vi "TImeThresholdLogic(SubVI).vi"(2 "Position":dbl[](array[numeric]), 3 "Bits":dbl[](array[numeric]), 4 "Buffer":dbl[][](array[numeric])) -> (0 "Data":dbl[][](array[numeric]))   [LabVIEW 2017]
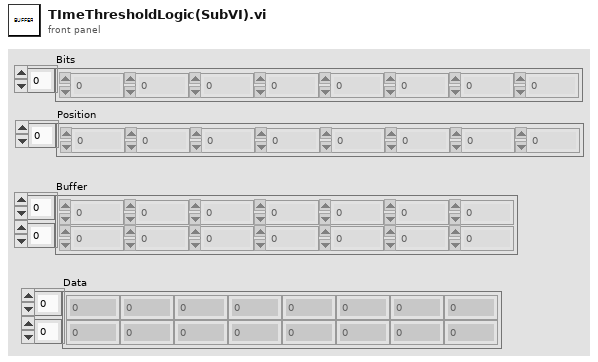
[diagram p1: front panel]
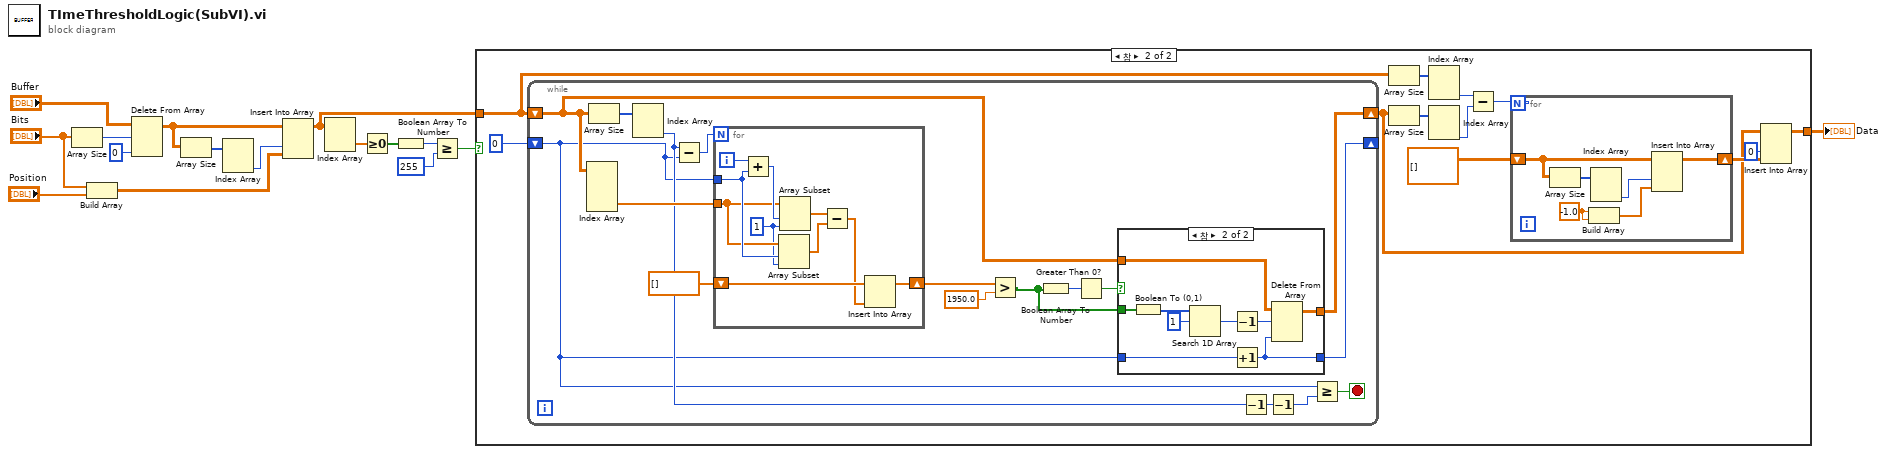
[diagram p0: block diagram]
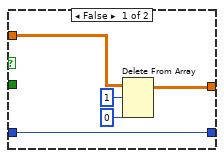
[diagram p3: hidden frame]
diagram:
  n1 = Array Size(array="Bits") -> (size(s)=w16:i32)
  n2 = Build Array("Bits", "Position") -> (w12:dbl[][])
  n3 = Delete From Array(array="Buffer", length=w16, index (col)=0 ("비활성화된 인덱스 (열)")) -> (array with subset deleted=w5:dbl[][])  [unwired: 1 in, 1 out]
  n4 = Array Size(array=w5) -> (size(s)=w11:i32[])
  n5 = Index Array(array=w11) -> (element #2=w10:i32)  [unwired: 2 in, 1 out]
  n6 = Insert Into Array(array=w5, index (col)=w10, new element=w12) -> (w4:dbl[][])  [unwired: 1 in]
  n7 = Index Array(array=w4) -> (element=w9:dbl[])  [unwired: 2 in]
  n8 = Greater Or Equal To 0?(x=w9) -> (x >= 0?=w8:bool[])
  n9 = Boolean Array To Number(Boolean array=w8) -> (number=w7:u32)
  n10 = Greater Or Equal?(x=w7, y=u32 255) -> (x >= y?=w3:bool)
  n11 = case shown="참" w3 {
    tunnel: w4 -> [w17 w28]
    tunnel: [w17 w18] -> w2
    frame False {
    }
    frame True {
      n12 = while {
        shift-right: [w46] -> _
        shift-left: 0 -> [w42]
        shift-right: [w41] -> w19
        shift-left: w28 -> [w45]
        stop <- w47 stop-if-true
        n13 = Index Array(array=w45) -> (element #2=w51:dbl[])  [unwired: 4 in, 1 out]
        n14 = Array Size(array=w45) -> (size(s)=w52:i32[])
        n15 = Index Array(array=w52) -> (element #2=w44:i32)  [unwired: 2 in, 1 out]
        n16 = Subtract(x=w44, y=w42) -> (x-y=w43:i32)
        n17 = for {
          N: w43 -> [_]
          tunnel: w51 -> [w73]
          tunnel: w42 -> [w74]
          shift-right: [w67] -> w38
          shift-left: dbl[] [] -> [w69]
          i -> [w76]
          w72 = 1 ("길이")
          n18 = Add(x=w76, y=w74) -> (x+y=w75:i32)
          n19 = Array Subset(array=w73, index=w74, length=w72) -> (w70:dbl[])
          n20 = Array Subset(array=w73, index=w75, length=w72) -> (w71:dbl[])
          n21 = Subtract(x=w71, y=w70) -> (x-y=w68:dbl[])
          n22 = Insert Into Array(array=w69, new element=w68) -> (w67:dbl[])  [unwired: 1 in]
        }
        n23 = Greater?(x=w38, y=1950.0) -> (0:w36:bool[])
        n24 = Boolean Array To Number(Boolean array=w36) -> (number=w49:u32)
        n25 = Greater Than 0?(x=w49) -> (x > 0?=w48:bool)
        n26 = case shown="참" w48 {
          tunnel: w36 -> [_ w66]
          tunnel: w42 -> [w53 w62]
          tunnel: w45 -> [w57 w61]
          tunnel: [w54 w60] -> w41
          tunnel: [w53 w59] -> w46
          frame False {
            n27 = Delete From Array(array=w57, length=1 ("길이"), index (col)=0 ("비활성화된 인덱스 (열)")) -> (array with subset deleted=w54:dbl[][])  [unwired: 1 in, 1 out]
          }
          frame True {
            n28 = Boolean To (0,1)(Boolean=w66) -> (0, 1=w58:i16[])
            n29 = Search 1D Array(1D array=w58, element=i16 1 ("원소")) -> (index of element=w64:i32)  [unwired: 1 in]
            n30 = Decrement(x=w64) -> (x-1=w63:i32)
            n31 = Increment(x=w62) -> (x+1=w59:i32)
            n32 = Delete From Array(array=w61, length=w63, index (col)=w59) -> (array with subset deleted=w60:dbl[][])  [unwired: 1 in, 1 out]
          }
        }
        n33 = Decrement(x=w44) -> (x-1=w40:i32)
        n34 = Decrement(x=w40) -> (x-1=w39:i32)
        n35 = Greater Or Equal?(x=w42, y=w39) -> (x >= y?=w47:bool)
      }
      n36 = Array Size(array=w28) -> (size(s)=w27:i32[])
      n37 = Array Size(array=w19) -> (size(s)=w26:i32[])
      n38 = Index Array(array=w27) -> (element #2=w25:i32)  [unwired: 2 in, 1 out]
      n39 = Index Array(array=w26) -> (element #2=w24:i32)  [unwired: 2 in, 1 out]
      n40 = Subtract(x=w25, y=w24) -> (x-y=w23:i32)
      n41 = for {
        N: w23 -> [_]
        shift-right: [w30] -> w21
        shift-left: dbl[][] [] -> [w35]
        w32 = -1.0 ("원소")
        n42 = Array Size(array=w35) -> (size(s)=w34:i32[])
        n43 = Build Array(w32, w32) -> (w31:dbl[])
        n44 = Index Array(array=w34) -> (element #2=w33:i32)  [unwired: 2 in, 1 out]
        n45 = Insert Into Array(array=w35, index (col)=w33, new element=w31) -> (w30:dbl[][])  [unwired: 1 in]
      }
      n46 = Insert Into Array(array=w19, index (col)=0 ("비활성화된 인덱스 (열)"), new element=w21) -> (w18:dbl[][])  [unwired: 1 in]
    }
  }
  "Data" <- w2
